vi "close.vi"(8 "error in (no error)":errorcluster, 11 "A66xxSupply in":refnum<class "A66xxSupply.lvclass">) -> (0 "error out":errorcluster)   [LabVIEW 2011, in "Hardware.lvlib" / "Channels.lvlib" / "A66xxSupply.lvclass"]
doc: "Closes the analog output device."
uses:
  A66xxSupply.lvclass
  AnalogOutput.lvclass
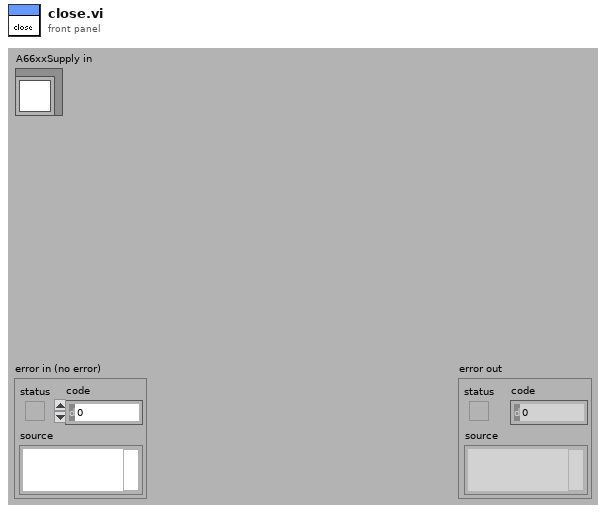
[diagram p1: front panel]
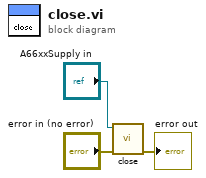
[diagram p0: block diagram]
diagram:
  n1 = call-parent "close.vi"("error in (no error)"="error in (no error)", "AnalogOutput in"="A66xxSupply in") -> ("error out"=→"error out":errorcluster)  [unwired: 9 in]
